vi "Get System Image (Folder).vi"(4 "File and Directory Blacklist":string[](array[string]), 5 "Encryption Passphrase":string, 6 "Overwrite (F)":bool, 7 "Restart Automatically (T)":bool=TRUE, 8 "error in (no error)":errorcluster, 9 "Installed Software Only (F)":bool, 10 "Destination Folder":path, 11 "Session in":refnum<k21>) -> (0 "error out":errorcluster, 3 "Session out":refnum<k21>)   [LabVIEW 2017, in "nisyscfg.lvlib"]
doc: "Creates a system image folder—a copy of the contents and software on a primary hard drive of a system. The image folder is edited if needed and the contents applied to a system to restore it to the state captured on the image."
uses:
  <vilib>/nisyscfg/nisyscfg.lvlib
panel:
  # "This VI is deprecated. Use the following VI instead:\n\nvi.lib\\nisyscfg\\Create System Image (Folder).vi"
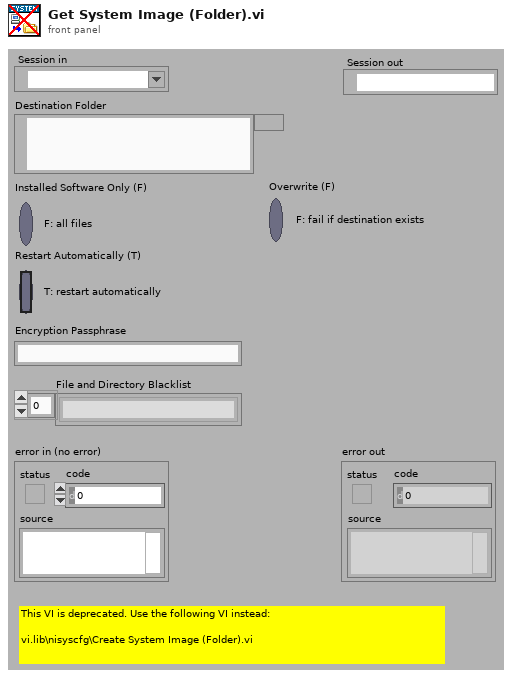
[diagram p1: front panel]
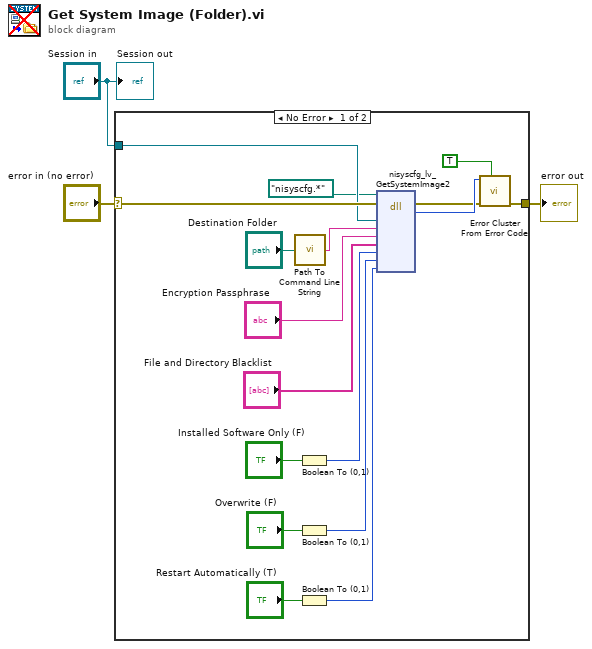
[diagram p0: block diagram]
diagram:
  n1 = case shown="No Error" "error in (no error)" {
    selector: "error in (no error)" -> [w16 w21]
    tunnel: [w20 w21] -> w3
    tunnel: "Session in" -> [w15 _]
    frame No Error {
      n2 = call <vilib>:"Path To Command Line String.vi"("path"="Destination Folder") -> ("string"=w4:string)
      n3 = Boolean To (0,1)(Boolean="Installed Software Only (F)") -> (0, 1=w17:i16)
      n4 = Boolean To (0,1)(Boolean="Overwrite (F)") -> (0, 1=w11:i16)
      n5 = Boolean To (0,1)(Boolean="Restart Automatically (T)") -> (0, 1=w8:i16)
      n6 = dll-call lib="nisyscfg.*" fn="nisyscfg_lv_GetSystemImage2" label="GetSystemImage"(path in=path "nisyscfg.*", error in=w16, "system"=w15, "localImagePath"=w4, "encryptionPassphrase"="Encryption Passphrase", "blacklist"="File and Directory Blacklist", "NISoftwareOnly"=w17, "overwriteIfExists"=w11, "restartAutomatically"=w8) -> (error out=w18:errorcluster, "result"=w19:i32)  [unwired: 8 in, 1 out]
      n7 = call <vilib>:"Error Cluster From Error Code.vi"("show call chain? (False)"=TRUE, "error in (no error)"=w18, "error code (0)"=w19) -> ("error out"=w20:errorcluster)  [unwired: 6 in]
    }
    frame Error {
    }
  }
  "error out" <- w3
  "Session out" <- "Session in"
